vi "Set Encoder.vi"(11 "IO Cluster In":T1={"Error"={"status"=FALSE, "code"=0, "source"=""}, "Encoder Calibration Values"=[22, 216], "Update Calibration"=FALSE, "JPEG Resolutions"=3, "Raw Resolutions"=1, "Image Mode"=enum."RAW Gray Scale", "FPGA Ref"=refnum} {"JPEG Resolutions" items=["160x128"=3, "320x240"=5, "640x480"=7]; "Raw Resolutions" items=["80x60"=1, "160x120"=3, "128x128"=9, "128x96"=11]}) -> (3 "IO Cluster Out":T1={"Error"={"status"=FALSE, "code"=0, "source"=""}, "Encoder Calibration Values"=[22, 216], "Update Calibration"=FALSE, "JPEG Resolutions"=3, "Raw Resolutions"=1, "Image Mode"=enum."RAW Gray Scale", "FPGA Ref"=refnum} {"JPEG Resolutions" items=["160x128"=3, "320x240"=5, "640x480"=7]; "Raw Resolutions" items=["80x60"=1, "160x120"=3, "128x128"=9, "128x96"=11]})   [LabVIEW 2018]
uses:
  QNET MS IO Cluster.ctl
  <vilib>/Utility/error.llb/Error Cluster From Error Code.vi
  <vilib>/rvi/errors/niLvFpgaAdjustHostInterfaceError.vi
  <vilib>/rvi/interface/nirviReadWriteControl/nirviReadWriteControl.xnode
  NiFpgaLv.dll
  <vilib>/rvi/interface/Simulation/niFpgaSimulationCallBeginRW.vi
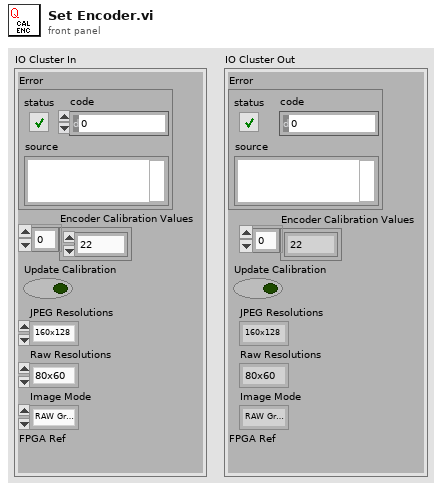
[diagram p1: front panel]
types:
  T1 = typedef "QNET MS IO Cluster.ctl" = cluster{"Error":errorcluster, "Encoder Calibration Values":i32[], "Update Calibration":bool, "JPEG Resolutions":u16, "Raw Resolutions":u16, "Image Mode":enum16{"RAW RGB", "RAW Gray Scale", "JPEG"}, "FPGA Ref":refnum<k20>}
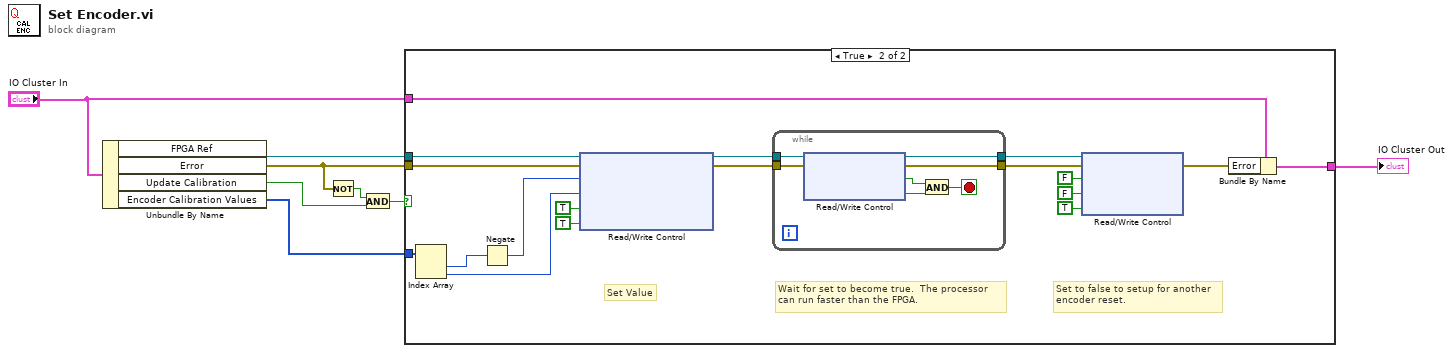
[diagram p0: block diagram]
diagram:
  n1 = Unbundle By Name("IO Cluster In") -> ("FPGA Ref"=w8:refnum<k20>, "Error"=w7:errorcluster, "Update Calibration"=w4:bool, "Encoder Calibration Values"=w3:i32[])
  n2 = Not(x=w7) -> (.not. x?=w6:bool)
  n3 = And(x=w6, y=w4) -> (x .and. y?=w5:bool)
  n4 = case shown="True" w5 {
    tunnel: [w9 w27] -> w1
    tunnel: "IO Cluster In" -> [w9 w26]
    tunnel: w8 -> [_ w23]
    tunnel: w3 -> [_ w13]
    tunnel: w7 -> [_ w12]
    frame False {
    }
    frame True {
      # "Set to false to setup for another\nencoder reset."
      # "Wait for set to become true.  The processor\ncan run faster than the FPGA."
      # "Set Value"
      n5 = Index Array(array=w13) -> (element #1=w15:i32, element #2=w14:i32)  [unwired: 2 in]
      n6 = Negate(x=w15) -> (-x=w10:i32)
      n7 = xnode "Read/Write Control"("FPGA VI Reference In"=w23, "error in"=w12, "Encoder 0 Reset Value"=w10, "Encoder 1 Reset Value"=w14, "Encoder 0 Reset"=TRUE, "Encoder 1 Reset"=TRUE) -> ("FPGA VI Reference Out"=w19:refnum<k20>, "error out"=w18:errorcluster)
      n8 = while {
        tunnel: w19 -> [w34]
        tunnel: [w32] -> w17
        tunnel: w18 -> [w33]
        tunnel: [w31] -> w16
        stop <- w28 stop-if-true
        n9 = xnode "Read/Write Control"("FPGA VI Reference In"=w34, "error in"=w33) -> ("FPGA VI Reference Out"=w32:refnum<k20>, "error out"=w31:errorcluster, "Encoder 0 Reset"=w29:bool, "Encoder 1 Reset"=w30:bool)
        n10 = And(x=w29, y=w30) -> (x .and. y?=w28:bool)
      }
      n11 = xnode "Read/Write Control"("FPGA VI Reference In"=w17, "error in"=w16, "Encoder 0 Reset"=FALSE, "Encoder 1 Reset"=FALSE, "Calibrated"=TRUE) -> ("error out"=w20:errorcluster)  [unwired: 1 out]
      n12 = Bundle By Name(cluster=w26, "Error"=w20) -> (w27:T1)
    }
  }
  "IO Cluster Out" <- w1
